vi "Incoming Bit.vi"(8 "error in (no error)":errorcluster, 10 "Set/Reset":bool, 11 "Controller -- Sig Acq Interface in":refnum<class "Controller -- Sig Acq Interface.lvclass">) -> (0 "error out":errorcluster, 3 "Controller -- Sig Acq Interface out":refnum<class "Controller -- Sig Acq Interface.lvclass">)   [LabVIEW 2022 SP3, in "Controller -- Signal Acq Interface.lvlib" / "Controller -- Sig Acq Interface.lvclass"]
uses:
  Controller -- Sig Acq Interface.lvclass
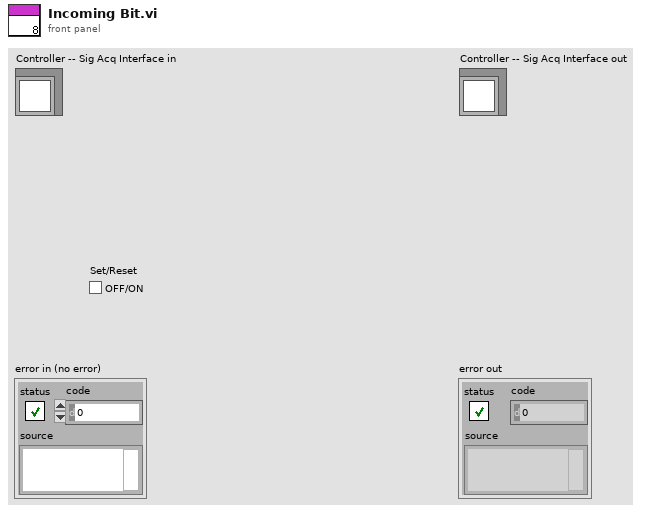
[diagram p1: front panel]
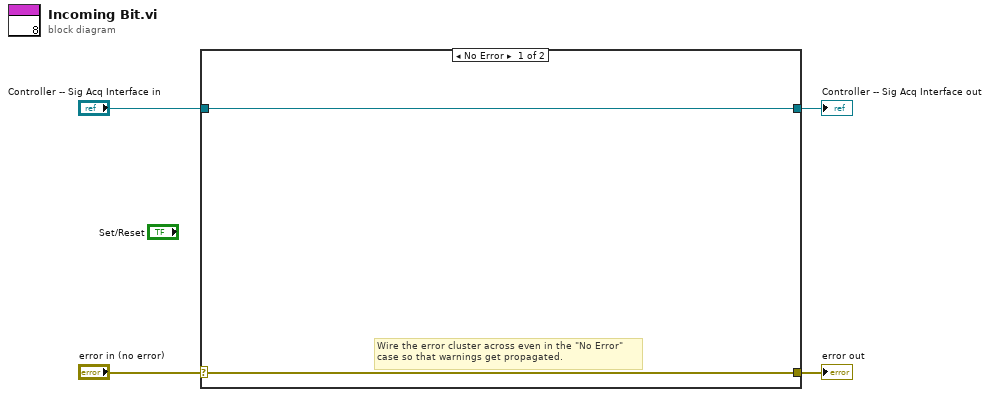
[diagram p0: block diagram]
diagram:
  n1 = case shown="No Error" "error in (no error)" {
    selector: "error in (no error)" -> [w6 w8]
    tunnel: [w6 w8] -> w3
    tunnel: [w5 w7] -> w1
    tunnel: "Controller -- Sig Acq Interface in" -> [w5 w7]
    frame No Error {
      # "Wire the error cluster across even in the \"No Error\"\ncase so that warnings get propagated."
    }
    frame Error {
    }
  }
  "error out" <- w3
  "Controller -- Sig Acq Interface out" <- w1
